vi "Laser Power Ctrl Index from Name.vi"(7 "Generic Class Ref":refnum<vi>) -> (8 "Index from Name":i32)   [LabVIEW 2016]
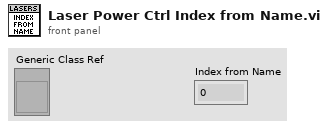
[diagram p1: front panel]
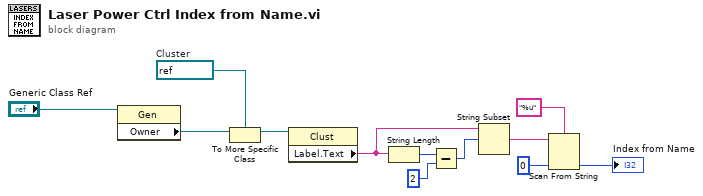
[diagram p0: block diagram]
diagram:
  w5 = refnum<vi> refnum  # Cluster
  n1 = property class="Gen"(reference="Generic Class Ref") -> ("Owner"=w4:refnum<vi>)  [unwired: 1 in, 2 out]
  n2 = To More Specific Class(target class=w5, reference=w4) -> (specific class reference=w6:refnum<vi>)  [unwired: 1 in, 1 out]
  n3 = property class="Clust"(reference=w6) -> ("Label.Text"=w3:string)  [unwired: 1 in, 2 out]
  n4 = String Length(string=w3) -> (length=w12:i32)
  n5 = Subtract(x=w12, y=2) -> (x-y=w10:i32)
  n6 = String Subset(string=w3, offset (0)=w10) -> (substring=w7:string)  [unwired: 1 in]
  n7 = Scan From String(format string="%u", input string=w7, default 1=0) -> (output 1=→"Index from Name":i32)  [unwired: 2 in, 3 out]
